vi "Set Plot Style.vi"(8 "error in (no error)":errorcluster, 9 "Plot Style":T1(ring), 10 "Channel":i32, 11 "Graph Manager in":refnum<class "Graph Manager.lvclass">) -> (0 "error out":errorcluster, 2 "Channel out":i32, 3 "Graph Manager out":refnum<class "Graph Manager.lvclass">)   [LabVIEW 2016, in "Graph Manager.lvclass"]
uses:
  Graph Manager.lvclass
  Graph Manager.lvclass/Graph Manager.ctl
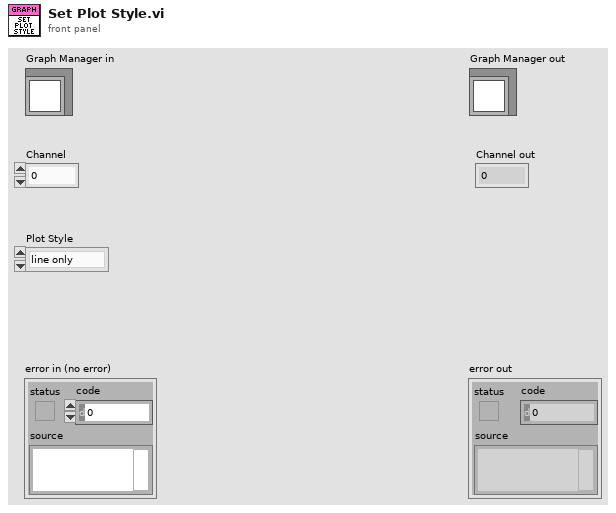
[diagram p1: front panel]
types:
  T1 = enum8{"line only", "points only", "points and lines", "none"}
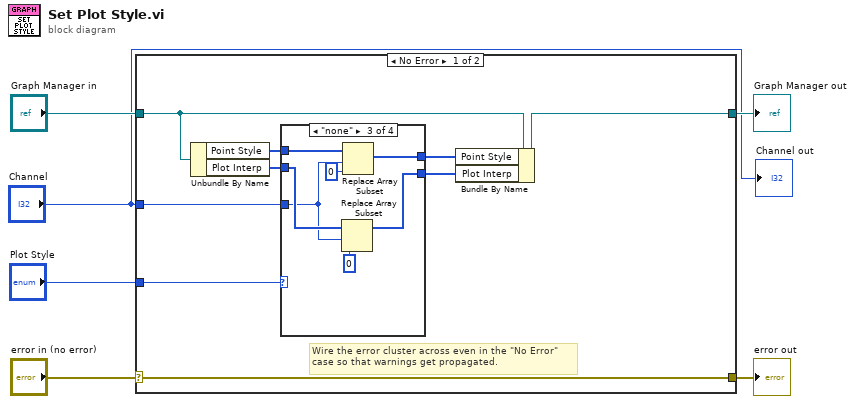
[diagram p0: block diagram]
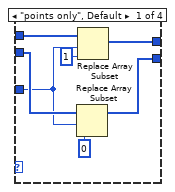
[diagram p2: hidden frame]
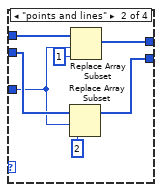
[diagram p3: hidden frame]
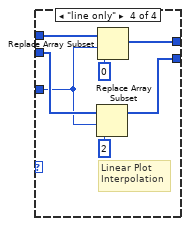
[diagram p4: hidden frame]
diagram:
  n1 = case shown="No Error" "error in (no error)" {
    selector: "error in (no error)" -> [w15 w45]
    tunnel: [w15 w45] -> w5
    tunnel: [w12 w44] -> w3
    tunnel: "Graph Manager in" -> [w13 w44]
    tunnel: "Channel" -> [w10 _]
    tunnel: "Plot Style" -> [w9 _]
    frame No Error {
      # "Wire the error cluster across even in the \"No Error\"\ncase so that warnings get propagated."
      n2 = Unbundle By Name(w13) -> ("Point Style"=w14:u8[], "Plot Interp"=w8:u8[])
      n3 = case shown="\"none\"" w9 {
        tunnel: w14 -> [w22 w29 w36 w43]
        tunnel: [w21 w28 w35 w42] -> w11
        tunnel: w10 -> [w18 w25 w32 w39]
        tunnel: w8 -> [w20 w27 w34 w41]
        tunnel: [w19 w26 w33 w40] -> w7
        frame "points only", Default {
          n4 = Replace Array Subset(array=w20, new element=u8 0 ("new element/subarray"), index=w18) -> (w19:u8[])
          n5 = Replace Array Subset(array=w22, new element=u8 1 ("new element/subarray"), index=w18) -> (w21:u8[])
        }
        frame "points and lines" {
          n6 = Replace Array Subset(array=w27, new element=u8 2 ("new element/subarray"), index=w25) -> (w26:u8[])
          n7 = Replace Array Subset(array=w29, new element=u8 1 ("new element/subarray"), index=w25) -> (w28:u8[])
        }
        frame "none" {
          n8 = Replace Array Subset(array=w34, new element=u8 0 ("new element/subarray"), index=w32) -> (w33:u8[])
          n9 = Replace Array Subset(array=w36, new element=u8 0 ("new element/subarray"), index=w32) -> (w35:u8[])
        }
        frame "line only" {
          # "Linear Plot\nInterpolation"
          n10 = Replace Array Subset(array=w41, new element=u8 2 ("new element/subarray"), index=w39) -> (w40:u8[])
          n11 = Replace Array Subset(array=w43, new element=u8 0 ("new element/subarray"), index=w39) -> (w42:u8[])
        }
      }
      n12 = Bundle By Name(cluster=w13, "Point Style"=w11, "Plot Interp"=w7) -> (w12:refnum<class "Graph Manager.lvclass">)
    }
    frame Error {
    }
  }
  "error out" <- w5
  "Graph Manager out" <- w3
  "Channel out" <- "Channel"
